vi "DefineVariableChoice.vi"() -> ()   [LabVIEW 2020]
panel:
  in  "Set":bool
  in  "Exit":bool
  in  "Add Choices":string
  in  "Choices":u16(ring) items=["numeric", "string", "1darray", "image", "on,off", "open,closed", "low,medium,high", "path", "outofrange,inrange", "1 mega ohm,50 ohms", "AC,DC,Ground", "Positive,Negative", "Field 1,Field2,Any Field,Any Line,Any Number", "AC,DC,HF Reject,LF Reject,AC Plus HF Reject", "Channel 0,Channel 1,External TRIG", "Entering,Leaving", "M-NTSC,B/G-PAL,SECAM,M-PAL,more", "Immediate,Analog Edge,Analog Window,Analog Hysteresis,Video,Digital Edge", "T0,T1,A,B,C,D,E,F,G,H", "Internal,External rising edges,External falling edges,Single shot external rising edges,Single shot external falling edges,Single shot,Line", "off,Triggers,AB,AB and CD,AB, CD and EF,AB, CD, EF and GH", "off,1,2,3,4,5,6,7,8,9", "T0,B,C,D", "T0,A,C,D", "T0,A,B,D", "T0,A,B,C", "TCPIP,Serial", "Not referenced,Referenced", "MZ switch and encoder Index,current position as HOME,MZ switch only,EoR- switch and encoder Index,EoR- switch only", "NOT REFERENCED,CONFIGURATION,HOMING,MOVING,READY,DISABLE,JOGGING", "High Z,50 Ohm", "TTL,NIM,ECL,VAR", "Internal,External,Single Shot,Burst,Line", "+ve edge,-ve edge", "Not referenced,Homing,Moving,Ready", "RTSI 0,RTSI 1,RTSI 2,RTSI 3,RTSI 4,RTSI 5,RTSI 6,PFI 0,PFI 1,PFI 2,PXI Star Trigger", "Continuous,Single Shot", "Not referenced,Homing,Moving,Ready", "Forward,Backward,Undefined", "pos,neg", "1,2,4,5,10", "TTL0,TTL1,TTL2,TTL3,TTL4,TTL5,TTL6,TTL7,ECL0,ECL1,Input Channel 1,Input Channel 2,Input Channel 3,Input Channel 4,External Trigger Source,STAR,Manual Trigger,Pattern", "1,2,3,4,5,6", "Diode,Low Power,High Power,undefined", "Error,Moving,OK", "n/a,max,min,energy", "Flipper,Plunger", "Remove,Insert", "IN,OUT", "Internal,External", "1f,3f,10f,30f,100f,300f,1p,3p,10p,30p,100p,300p,1n,3n,10n,30n,100n,300n,1u,3u,10u,30u,100u,300u,1m,3m,10m,30m,100m,300m,1,3,10,30,100,300,1k,3k,10k,30k,100k,300k,1M,3M,10M,30M,100M,300M", "yes,no", "IS_SET_TRIG_OFF,IS_SET_TRIG_HI_LO,IS_SET_TRIG_LO_HI,IS_SET_TRIG_SOFTWARE,IS_GET_EXTERNAL_TRIGGER,IS_GET_TRIGGER_STATUS", "Disable,High,Low", "64,128,256,512", "Moving/Unknown,OD1,OD2,OD3,OD4,OD5,Open(6)", "temporal CAM,spatial CAM", "out,in,Unknown", "Channel0,Channel1,Channel2,Channel3,Channel4,Channel5,Channel6,Channel7,n/a", "n/a,max,min,energy,trigger,maxtime,mintime,mean", "absolute,gauge", "1p,3p,10p,30p,100p,300p,1n,3n,10n,30n,100n,300n,1u,3u,10u,30u,100u,300u,1m,3m,10m,30m,100m,300m,1,3,10,30,100,300,1k,3k,10k,30k,100k,300k,1meg,3meg,10meg,30meg,100meg,300meg", "Internal 1,Internal 2,External,SS1,SS2,SSExt,LSS,OFF", "off,on,reset,fault", "Double,Boolean", "n/a,max,min,energy,trigger,maxtime,mintime,mean", "FL1-f8x08,FL1-f8x06,FL1-f8,ch300-f50,FL2G-f8,FL3M14-f8,FL3M14-f8x08,FL3M14-f8x08(2x2)", "Serial,TCP", "Pressure,Flow", "Numeric,String", "N/A,Free Run/Timed,Trigger First (PM only),Ext Sync/Strobed,Variable Exp (PM only),Flash Mode (PM only)", "Software,Hardware", "Immediate,Analog Edge", "Channel1,Channel2,Channel3,Channel4,AC Line,Aux", "DC,HF Reject,LF Reject,Noise Reject,AC", "Rising,Falling", "1E+3,10E+3,100E+3,1E+6,5E+6,10E+6", "1M,75,50", "FULL,250 MHz, 150 MHz, 20 MHz", "Channel 1,Channel 2,Channel 3,Channel 4,Math,Reference 1,Reference 2,Reference 3,Reference 4,Bus 1,Bus 2", "10KOhm,50Ohms", "Rising,Falling,Internal 80Mhz,Internal DSS,Remote,Disable", "Direct,Inverted", "Null,A,B,C,D,Trigger", "Auto,Manual", "J,K,N,R,S,T,B,E", "Deg C,Deg F,Kelvins,Deg R,From Custom Scale", "Built-In,Constant Value,Channel", "1f,3f,10f,30f,100f,300f,1p,3p,10p,30p,100p,300p,1n,3n,10n,30n,100n,300n,1u,3u,10u,30u,100u,300u,1m,3m,10m,30m,100m,300m,1,3,10,30,100,300,1K,3K,10K,30K,100K,300K,1M,3M,10M,30M,100M,300M", "left,right", "on demand,continuous,scan", "1,2,3,4", "50,100,250,500,1000,2500,5K,10K,25K,50K,100K,250K,500K,1M,2M,2.5M,5M,10M,25M,50M,100M", "Full,20MHZ,25MHZ,200MHZ,250MHZ,1GHZ,3GHZ,4GHZ", "Channel 1,Channel 2,Channel 3,Channel 4,External,Power Line", "Auto,Normal,Single,Single, auto trigger", "A1M,D1M,D50,Ground,DC,AC", "POS (+),NEG (-)", "HOME,POS (+),NEG (-)", "Idel,Moving,L- (neg limit),L+ (pos limit),Homed", "HOME,POS (+),NEG (-),none", "HOME,POS (+),NEG (-),done", "Full,20MHZ,200MHZ", "Full,25MHZ,20MHZ,200MHZ", "HOME,done", "Idel,Moving,Accelerating,Decelerating,L- (neg limit),L+ (pos limit),Homed", "homing,limiting,done", "true,false", "default,inverted", "choice", "Enable,Disable", "4J,8J", "50usec,100usec", "Energy,Power", "Removed,Inserted,Unknown,Moving", "20.00J,4.00J,400mJ,40.0mJ,4.00mJ", "50uS,1.0mS", "248,355,532,800,2940,193", "Auto,Normal,Single,Single auto trigger", "Voltage,Current", "PNG,BMP,JPEG,TDMS", "PNG,BMP,JPEG,TDMS,hdf5", "FL1-f8x08,FL1-f8x06,FL1-f8,ch300-f50,FL2G-f8,FL3M14-f8,FL3M14-f8x08,FL3M14-f8x08(2x2),aca720-f8,aca1440-f8", "10 mV, 20mV, 50mV, 100mV, 200mV, 500mV, 1V, 2V, 5V, 10V, 20V"]
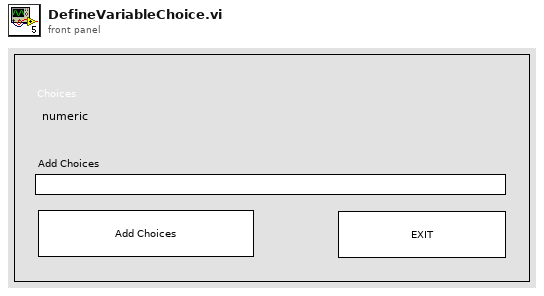
[diagram p1: front panel]
types:
  T1 = enum32{"Invalid", "Standard", "Closed", "Hidden", "Minimized", "Maximized"}
  T2 = enum32{"invalid app kind", "Development System", "Run Time System", "Student Edition", "Embedded LabVIEW", "Evaluation", "Custom"}
  T3 = typedef "mysql_authentication.ctl" = cluster{"User":string, "Password":string, "Database":string}
  T4 = cluster{"Core":cluster{"Current VI Reference":refnum<vi>, "Close Panel on Exit?":bool}, "SQL Server Info":cluster{"Port":u16, "IP Address":string, "Authentication":T3}, "Your string data":string}
  T5 = cluster{"Port":u16, "IP Address":string, "Authentication":T3}
  T6 = cluster{"Current VI Reference":refnum<vi>, "Close Panel on Exit?":bool}
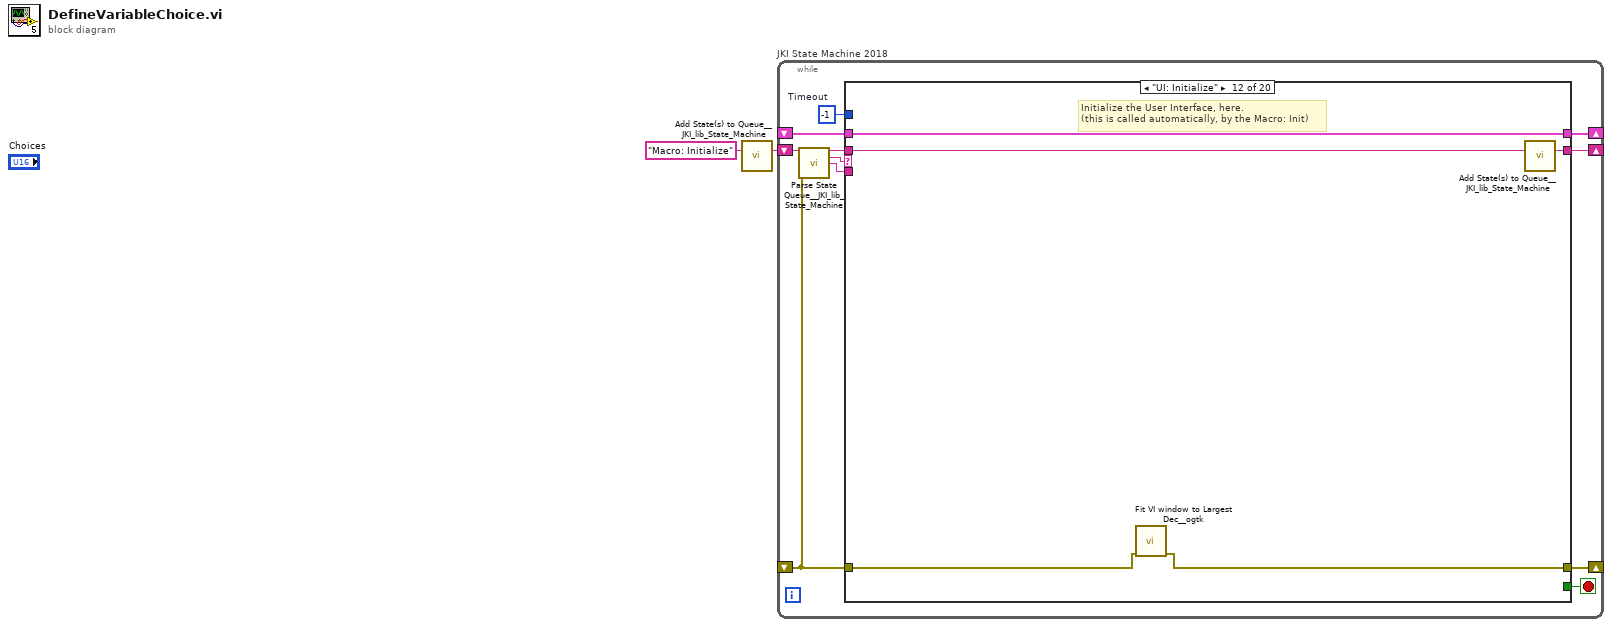
[diagram p0: block diagram]
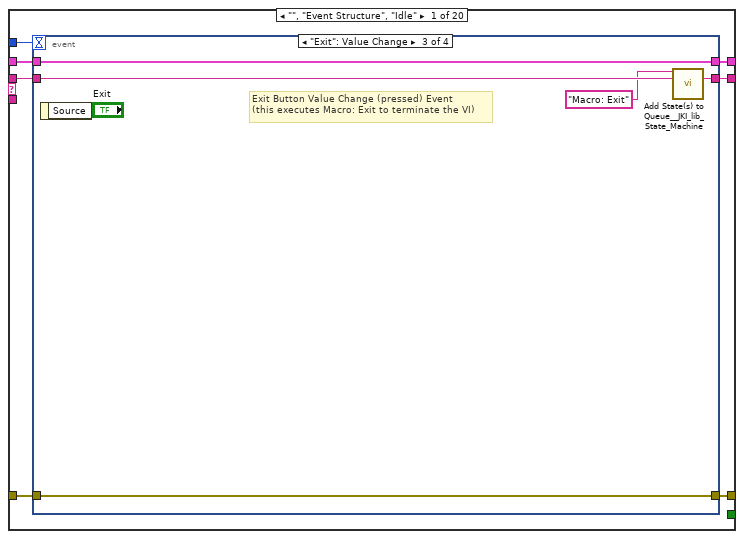
[diagram p2: hidden frame]
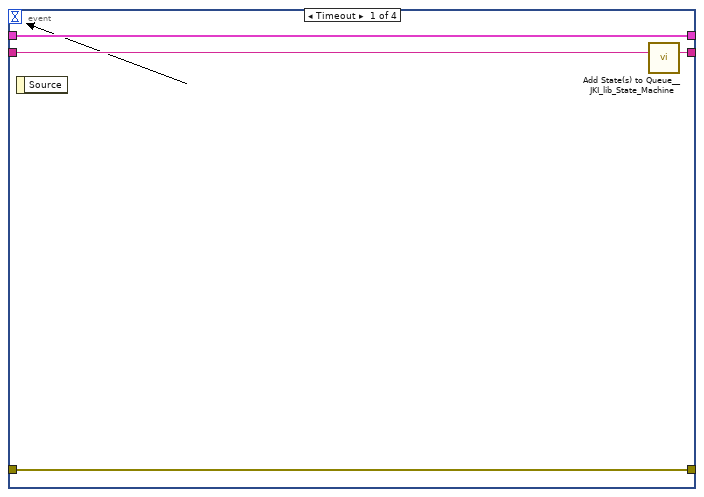
[diagram p3: hidden frame]
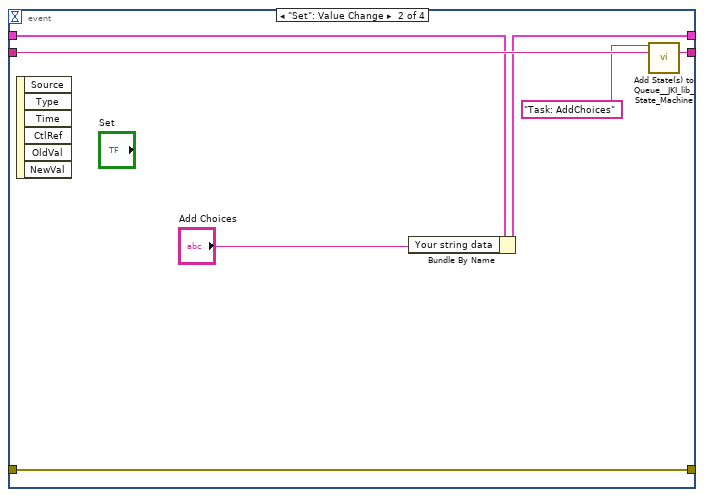
[diagram p4: hidden frame]
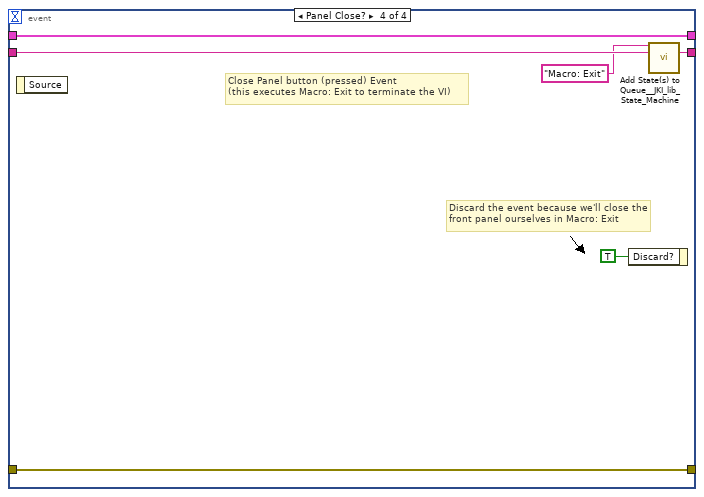
[diagram p5: hidden frame]
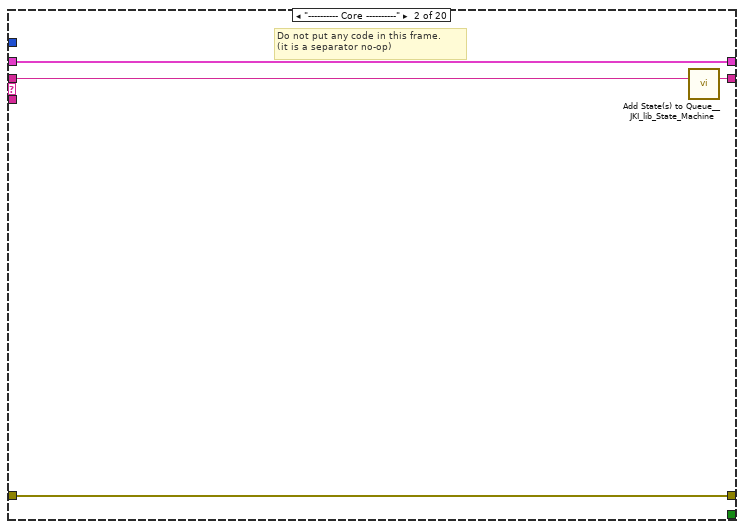
[diagram p6: hidden frame]
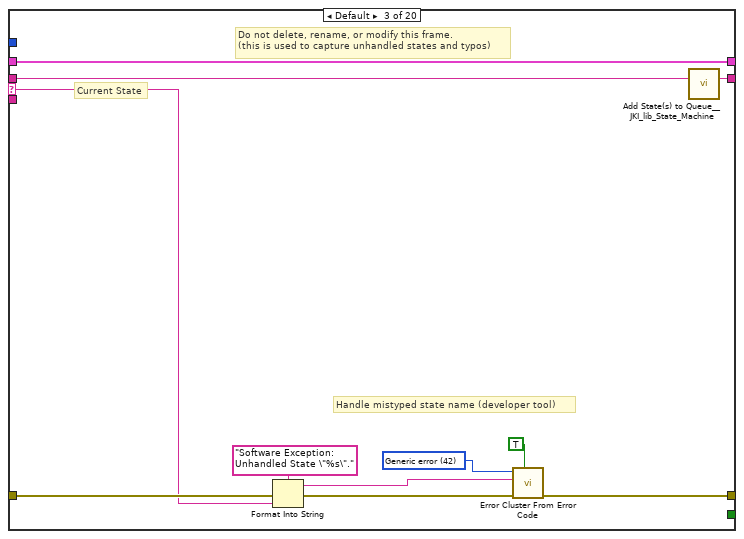
[diagram p7: hidden frame]
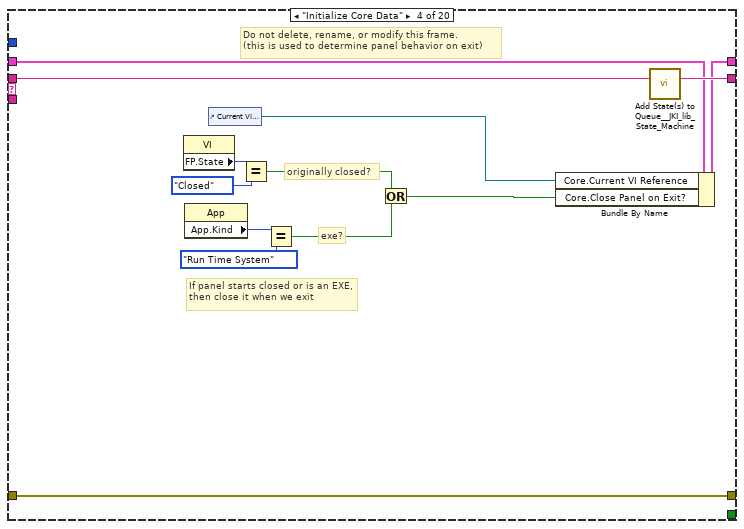
[diagram p8: hidden frame]
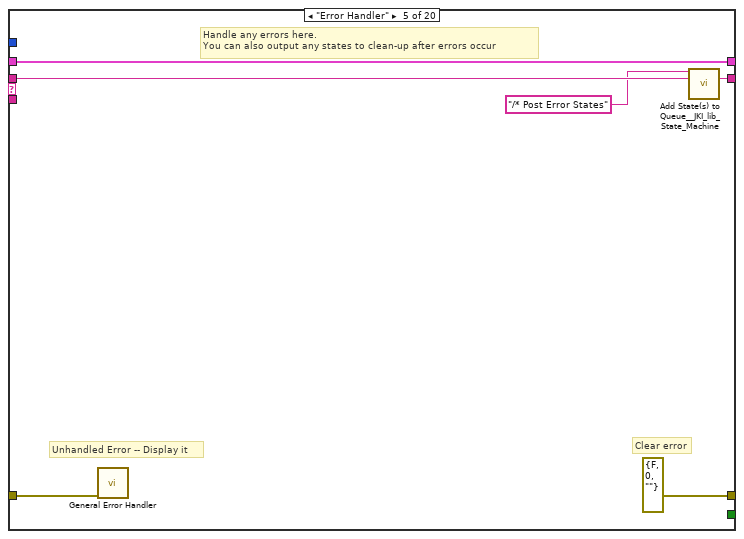
[diagram p9: hidden frame]
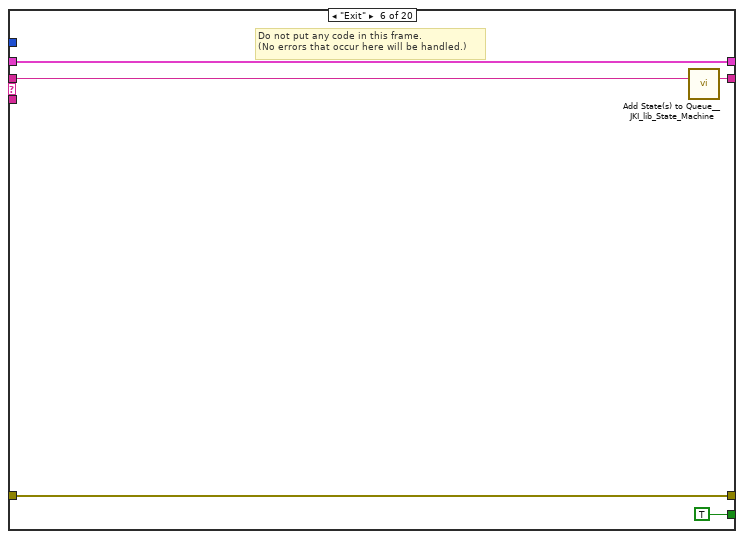
[diagram p10: hidden frame]
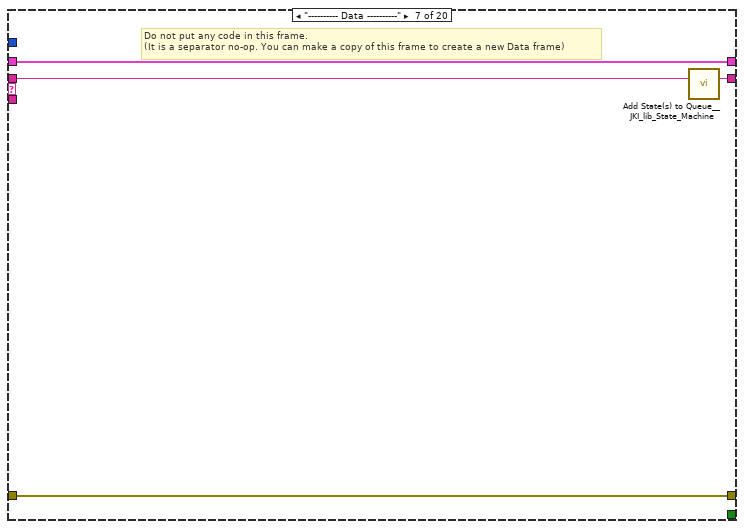
[diagram p11: hidden frame]
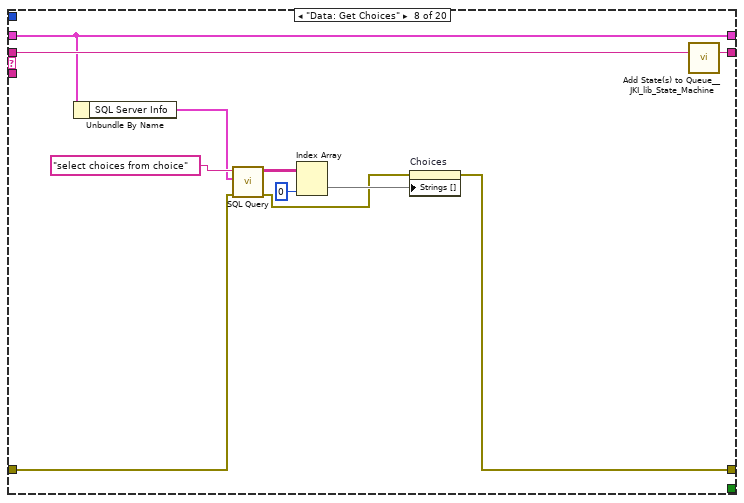
[diagram p12: hidden frame]
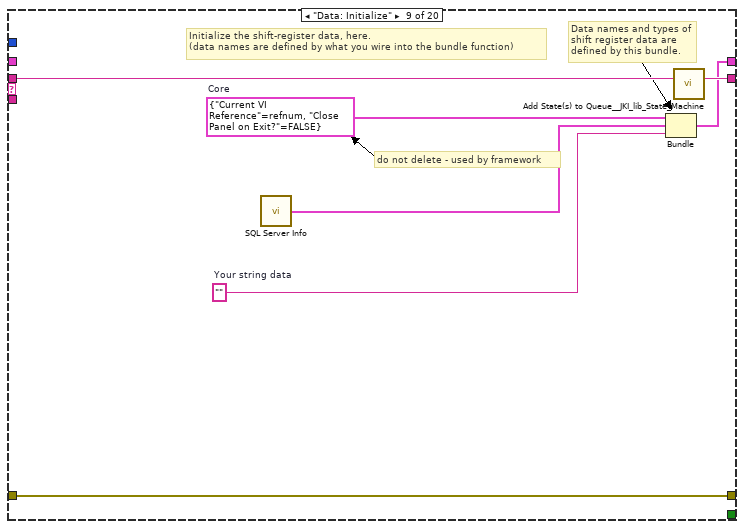
[diagram p13: hidden frame]
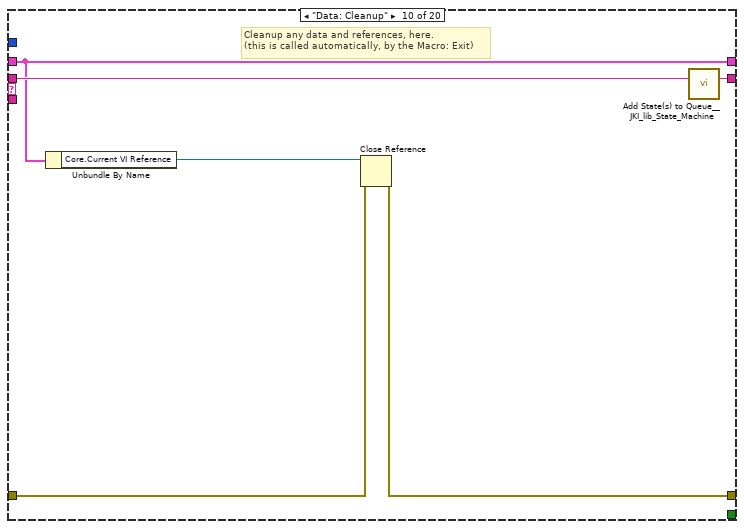
[diagram p14: hidden frame]
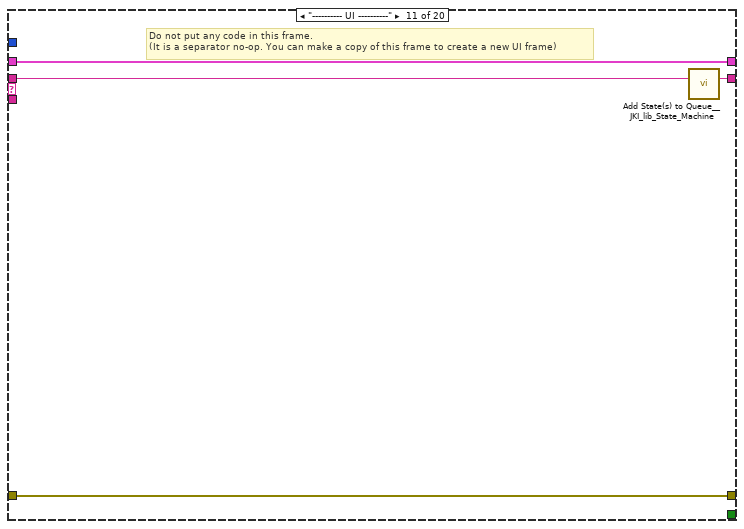
[diagram p15: hidden frame]
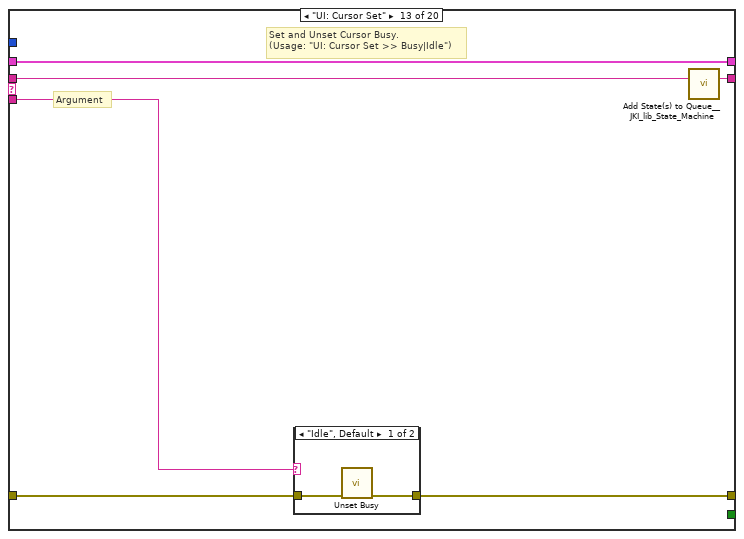
[diagram p16: hidden frame]
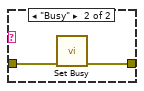
[diagram p17: hidden frame]
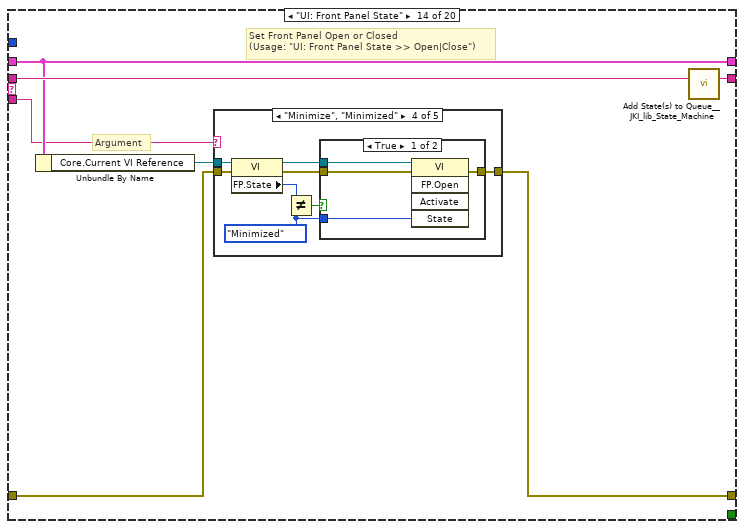
[diagram p18: hidden frame]
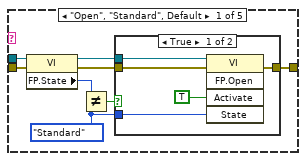
[diagram p19: hidden frame]
diagram:
  n1 = call <vilib>:"Add State(s) to Queue__JKI_lib_State_Machine.vi"("State(s) in (\"\")"="Macro: Initialize") -> ("States Out"=w2:string)  [unwired: 14 in]
  n2 = while "JKI State Machine 2018" {
    shift-right: [w6] -> _
    shift-left: _ -> [w5]
    shift-right: [w9] -> _
    shift-left: _ -> [w3]
    shift-right: [w8] -> _
    shift-left: w2 -> [w10]
    stop <- w7 stop-if-true
    w4 = -1  # Timeout
    n3 = call <vilib>:"Parse State Queue__JKI_lib_State_Machine.vi"("State Queue"=w10, "Error In (no error)"=w3) -> ("Remaining States"=w12:string, "Current State"=w13:string, "Arguments"=w11:string)  [unwired: 11 in]
    n4 = case shown="\"UI: Initialize\"" w13 {
      selector: w13 -> [_ _ w47 _ _ _ _ _ _ _ _ _ _ _ _ _ _ _ _ _]
      tunnel: w12 -> [w20 w46 w51 w70 w76 w81 w85 w96 w103 w109 w113 w118 w124 w135 w204 w209 w219 w223 w234 w238]
      tunnel: w11 -> [_ _ _ _ _ _ _ _ _ _ _ _ w119 w129 _ _ _ _ _ _]
      tunnel: w5 -> [w18 w43 w49 w63 w73 w79 w82 w94 _ w104 w110 w116 w122 w131 w201 w206 w216 w220 w229 w235]
      tunnel: [w17 w44 w53 w67 errorcluster {"status"=FALSE, "code"=0, "source"=""} ("error out") w78 w83 w86 w100 w105 w111 w115 w120 w132 w202 w207 w217 w221 w225 w236] -> w9
      tunnel: w3 -> [w16 w44 w52 w67 w72 w78 w83 w88 w100 w106 w111 w114 w121 w133 w202 w207 w217 w221 w224 w236]
      tunnel: [w19 w45 w50 w69 w75 w80 w84 w95 w102 w108 w112 w117 w123 w134 w203 w208 w218 w222 w233 w237] -> w8
      tunnel: [_ _ _ _ _ TRUE _ _ _ _ _ _ _ _ _ _ _ _ _ _] -> w7
      tunnel: [w15 w43 w49 w68 w73 w79 w82 w94 w101 w104 w110 w116 w122 w131 w201 w206 w216 w220 w229 w235] -> w6
      tunnel: w4 -> [w14 _ _ _ _ _ _ _ _ _ _ _ _ _ _ _ _ _ _ _]
      frame "", "Event Structure", "Idle" {
        n5 = event shown="[2] \"Exit\": Value Change" {
          selector: _ -> [_ _ _ _]
          dyn-events: _ -> [_ _ _ _]
          timeout: w14 -> [_ _ _ _]
          tunnel: w20 -> [w24 w31 w36 w42]
          tunnel: [w23 w30 w35 w41] -> w19
          tunnel: w18 -> [w21 w28 w33 w39]
          tunnel: [w22 w29 w34 w40] -> w17
          tunnel: w16 -> [w22 w29 w34 w40]
          tunnel: [w21 w27 w33 w39] -> w15
          event Timeout {
            n6 = event-data() -> ()  [unwired: 1 in, 1 out]
            n7 = call <vilib>:"Add State(s) to Queue__JKI_lib_State_Machine.vi"("State(s) in (\"\")"=w24) -> ("States Out"=w23:string)  [unwired: 14 in]
          }
          event "Set": Value Change {
            n8 = event-data() -> ()  [unwired: 1 in, 6 out]
            n9 = Bundle By Name(cluster=w28, "Your string data"="Add Choices") -> (w27:T4)
            n10 = call <vilib>:"Add State(s) to Queue__JKI_lib_State_Machine.vi"("State(s) in Front (\"\")"="Task: AddChoices" ("State(s) in Front (\"\")"), "State(s) in (\"\")"=w31) -> ("States Out"=w30:string)  [unwired: 13 in]
          }
          event "Exit": Value Change {
            # "Exit Button Value Change (pressed) Event\n(this executes Macro: Exit to terminate the VI)"
            n11 = event-data() -> ()  [unwired: 1 in, 1 out]
            n12 = call <vilib>:"Add State(s) to Queue__JKI_lib_State_Machine.vi"("State(s) in Front (\"\")"="Macro: Exit", "State(s) in (\"\")"=w36) -> ("States Out"=w35:string)  [unwired: 13 in]
          }
          event Panel Close? {
            # "Discard the event because we'll close the front panel ourselves in Macro: Exit"
            # "Close Panel button (pressed) Event\n(this executes Macro: Exit to terminate the VI)"
            n13 = event-data() -> ()  [unwired: 1 in, 1 out]
            n14 = event-data("Discard?"=TRUE) -> ()  [unwired: 1 in, 1 out]
            n15 = call <vilib>:"Add State(s) to Queue__JKI_lib_State_Machine.vi"("State(s) in Front (\"\")"="Macro: Exit", "State(s) in (\"\")"=w42) -> ("States Out"=w41:string)  [unwired: 13 in]
          }
        }
      }
      frame "---------- Core ----------" {
        # "Do not put any code in this frame.\n(it is a separator no-op)"
        n16 = call <vilib>:"Add State(s) to Queue__JKI_lib_State_Machine.vi"("State(s) in (\"\")"=w46) -> ("States Out"=w45:string)  [unwired: 14 in]
      }
      frame Default {
        w56 = 42 items=["No error", "Argument error", "Memory is full", "Out of zone", "End of file", "File already open", "Generic file I/O error", "File not found", "File permission error", "Disk is full", "Duplicate path", "Too many files open", "System feature not enabled", "Resource file not found", "Cannot add resource", "Resource not found", "Image not found", "Image memory error", "Pen does not exist", "Config type invalid", "Config token not found", "Config parse error", "Config memory error", "Bad external code format", "Bad external code offset", "External code not present", "Null window", "Destroy window error", "Null menu", "Print aborted", "Bad print record", "Print driver error", "Windows error during printing", "Memory error during printing", "Print dialog error", "Generic print error", "Invalid device refnum", "Device not found", "Device parameter error", "Device unit error", "Cannot open device", "Device call aborted", "Generic error", "Cancelled by user", "Object ID too low", "Object ID too high", "Object not in heap", "Unknown heap", "Unknown object (invalid DefProc)", "Unknown object (DefProc not in table)", "Message out of range", "Invalid (null) method", "Unknown message", "Manager call not supported", "Bad address", "Network operation in progress", "Network operation timed out", "Connection is busy", "Network attribute not supported", "Network error", "Address in use", "System out of memory", "Connection aborted", "Connection refused", "Not connected", "Already connected", "Connection closed", "Initialization error (interapplication manager)", "Bad occurrence", "Wait on unbound occurrence handler", "Occurrence queue overflow", "Datalog type conflict", "Unused", "Unrecognized type (interapplication manager)", "Memory corrupt", "Failed to make temporary DLL", "Old CIN version", "Drag socket not found", "Failed to load drop-object", "Failed to register OLE object", "Failed to release OLE object", "Format specifier type mismatch", "Unknown format specifier", "Too few format specifiers", "Too many format specifiers", "Scan failed", "Newer CIN version", "Error converting to variant", "Runtime menu error", "Password tampered", "Variant attribute not found", "Incompatible variant data type", "Event data is not available", "Event Store is not present", "Occurrence is not found", "Event Queue is not created", "Event info is not available", "Refnum passed is NULL", "Error retrieving Class GUID", "Error retrieving CoClass GUID", "Error retrieving TypeLib GUID.", "Bad built application magic bytes.", "Specific driver is different from the specific driver associated with the Logical Name.", "There is no session opened to the class driver.", "Max Error", "MAX - Error with config objects", "MAX - Error loading configuration", "MAX - Group not supported"]
        # "Current State"
        # "Do not delete, rename, or modify this frame.\n(this is used to capture unhandled states and typos)"
        # "Handle mistyped state name (developer tool)"
        n17 = Format Into String(format string="Software Exception: Unhandled State \"%s\"." ("message"), error in=w52, w47) -> (resulting string=w55:string, error out=w54:errorcluster)  [unwired: 1 in]
        n18 = call <vilib>:"Error Cluster From Error Code.vi"("show call chain? (False)"=TRUE, "error in (no error)"=w54, "error message (\"\")"=w55, "error code (0)"=w56) -> ("error out"=w53:errorcluster)  [unwired: 5 in]
        n19 = call <vilib>:"Add State(s) to Queue__JKI_lib_State_Machine.vi"("State(s) in (\"\")"=w51) -> ("States Out"=w50:string)  [unwired: 14 in]
      }
      frame "Initialize Core Data" {
        # "Do not delete, rename, or modify this frame.\n(this is used to determine panel behavior on exit)"
        # "originally closed?"
        # "exe?"
        # "If panel starts closed or is an EXE, then close it when we exit"
        n20 = property class="VI"() -> ("FP.State"=w60:T1)  [unwired: 2 in, 2 out]
        n21 = property class="App"() -> ("App.Kind"=w66:T2)  [unwired: 2 in, 2 out]
        n22 = control-ref of="Current VI Reference"() -> (w61:refnum<vi>)
        n23 = Equal?(x=w60, y=T1."Closed" ("Front Panel Window:State")) -> (x = y?=w58:bool)
        n24 = Equal?(x=w66, y=T2."Run Time System" ("Application:Kind")) -> (x = y?=w64:bool)
        n25 = Or(x=w58, y=w64) -> (x .or. y?=w62:bool)
        n26 = Bundle By Name(cluster=w63, "Core.Current VI Reference"=w61, "Core.Close Panel on Exit?"=w62) -> (w68:T4)
        n27 = call <vilib>:"Add State(s) to Queue__JKI_lib_State_Machine.vi"("State(s) in (\"\")"=w70) -> ("States Out"=w69:string)  [unwired: 14 in]
      }
      frame "Error Handler" {
        # "Unhandled Error -- Display it"
        # "Handle any errors here.\nYou can also output any states to clean-up after errors occur"
        # "Clear error"
        n28 = call <vilib>:"General Error Handler.vi"("error in (no error)"=w72) -> ()  [unwired: 10 in, 5 out]
        n29 = call <vilib>:"Add State(s) to Queue__JKI_lib_State_Machine.vi"("State(s) in Front (\"\")"="/* Post Error States", "State(s) in (\"\")"=w76) -> ("States Out"=w75:string)  [unwired: 13 in]
      }
      frame "Exit" {
        # "Do not put any code in this frame.\n(No errors that occur here will be handled.)"
        n30 = call <vilib>:"Add State(s) to Queue__JKI_lib_State_Machine.vi"("State(s) in (\"\")"=w81) -> ("States Out"=w80:string)  [unwired: 14 in]
      }
      frame "---------- Data ----------" {
        # "Do not put any code in this frame.\n(It is a separator no-op. You can make a copy of this frame to create a new Data frame)"
        n31 = call <vilib>:"Add State(s) to Queue__JKI_lib_State_Machine.vi"("State(s) in (\"\")"=w85) -> ("States Out"=w84:string)  [unwired: 14 in]
      }
      frame "Data: Get Choices" {
        n32 = Unbundle By Name(w94) -> ("SQL Server Info"=w89:T5)
        n33 = call "SQL Query.vi"("error in (no error)"=w88, "SQL Server Info"=w89, "Query"="select choices from choice") -> ("error out"=w87:errorcluster, "data"=w92:string[][])  [unwired: 7 in]
        n34 = Index Array(array=w92, index (col)=0 ("disabled index (col)")) -> (element=w93:string[])  [unwired: 1 in]
        n35 = property on="Choices" class="Ring (strict)"(error in=w87, "Strings []"=w93) -> (error out=w86:errorcluster)  [unwired: 1 in, 1 out]
        n36 = call <vilib>:"Add State(s) to Queue__JKI_lib_State_Machine.vi"("State(s) in (\"\")"=w96) -> ("States Out"=w95:string)  [unwired: 14 in]
      }
      frame "Data: Initialize" {
        w98 = T6 {"Current VI Reference"=refnum, "Close Panel on Exit?"=FALSE}  # Core
        w99 = ""  # Your string data
        # "do not delete - used by framework"
        # "Data names and types of shift register data are defined by this bundle."
        # "Initialize the shift-register data, here.\n(data names are defined by what you wire into the bundle function)"
        n37 = call "SQL Server Info.vi"() -> ("SQL Server Info"=w97:T5)
        n38 = Bundle("Core"=w98, "SQL Server Info"=w97, "Your string data"=w99) -> (w101:T4)  [unwired: 1 in]
        n39 = call <vilib>:"Add State(s) to Queue__JKI_lib_State_Machine.vi"("State(s) in (\"\")"=w103) -> ("States Out"=w102:string)  [unwired: 14 in]
      }
      frame "Data: Cleanup" {
        # "Cleanup any data and references, here.\n(this is called automatically, by the Macro: Exit)"
        n40 = Unbundle By Name(w104) -> ("Core.Current VI Reference"=w107:refnum<vi>)
        n41 = Close Reference(reference=w107, error in (no error)=w106) -> (error out=w105:errorcluster)
        n42 = call <vilib>:"Add State(s) to Queue__JKI_lib_State_Machine.vi"("State(s) in (\"\")"=w109) -> ("States Out"=w108:string)  [unwired: 14 in]
      }
      frame "---------- UI ----------" {
        # "Do not put any code in this frame.\n(It is a separator no-op. You can make a copy of this frame to create a new UI frame)"
        n43 = call <vilib>:"Add State(s) to Queue__JKI_lib_State_Machine.vi"("State(s) in (\"\")"=w113) -> ("States Out"=w112:string)  [unwired: 14 in]
      }
      frame "UI: Initialize" {
        # "Initialize the User Interface, here.\n(this is called automatically, by the Macro: Init)"
        n44 = call <userlib>:"Fit VI window to Largest Dec__ogtk.vi"("error in (no error)"=w114) -> ("error out"=w115:errorcluster)  [unwired: 5 in, 1 out]
        n45 = call <vilib>:"Add State(s) to Queue__JKI_lib_State_Machine.vi"("State(s) in (\"\")"=w118) -> ("States Out"=w117:string)  [unwired: 14 in]
      }
      frame "UI: Cursor Set" {
        # "Argument"
        # "Set and Unset Cursor Busy.\n(Usage: \"UI: Cursor Set >> Busy|Idle\")"
        n46 = case shown="\"Idle\", Default" w119 {
          tunnel: w121 -> [w126 w128]
          tunnel: [w125 w127] -> w120
          frame "Idle", Default {
            n47 = call <vilib>:"Unset Busy.vi"("error in (no error)"=w126) -> ("error out"=w125:errorcluster)  [unwired: 10 in]
          }
          frame "Busy" {
            n48 = call <vilib>:"Set Busy.vi"("error in (no error)"=w128) -> ("error out"=w127:errorcluster)  [unwired: 9 in, 1 out]
          }
        }
        n49 = call <vilib>:"Add State(s) to Queue__JKI_lib_State_Machine.vi"("State(s) in (\"\")"=w124) -> ("States Out"=w123:string)  [unwired: 14 in]
      }
      frame "UI: Front Panel State" {
        # "Argument"
        # "Set Front Panel Open or Closed\n(Usage: \"UI: Front Panel State >> Open|Close\")"
        n50 = Unbundle By Name(w131) -> ("Core.Current VI Reference"=w130:refnum<vi>)
        n51 = case shown="\"Minimize\", \"Minimized\"" w129 {
          tunnel: w133 -> [w141 w156 w167 w180 w193]
          tunnel: [w143 w157 w169 w182 w195] -> w132
          tunnel: w130 -> [w142 w154 w168 w181 w194]
          frame "Open", "Standard", Default {
            w136 = T1."Standard" ("State")
            n52 = property class="VI"(reference=w142, error in=w141) -> (reference out=w139:refnum<vi>, error out=w140:errorcluster, "FP.State"=w138:T1)
            n53 = Not Equal?(x=w138, y=w136) -> (x != y?=w137:bool)
            n54 = case shown="True" w137 {
              tunnel: [w147 w149] -> w143
              tunnel: w140 -> [w146 w149]
              tunnel: w139 -> [w145 _]
              tunnel: w136 -> [w144 _]
              frame True {
                n55 = invoke class="VI" method="FP.Open"(reference=w145, error in=w146, "Activate"=TRUE, "State"=w144) -> (error out=w147:errorcluster)  [unwired: 1 in, 4 out]
              }
              frame False {
              }
            }
          }
          frame "Close", "Closed" {
            n56 = property class="VI"(reference=w154, error in=w156) -> (reference out=w153:refnum<vi>, error out=w155:errorcluster, "FP.State"=w151:T1)
            n57 = Not Equal?(x=w151, y=T1."Closed" ("Front Panel Window:State")) -> (x != y?=w150:bool)
            n58 = case shown="True" w150 {
              tunnel: [w158 w161] -> w157
              tunnel: w155 -> [w158 w160]
              tunnel: w153 -> [_ w159]
              frame False {
              }
              frame True {
                n59 = invoke class="VI" method="FP.Close"(reference=w159, error in=w160) -> (error out=w161:errorcluster)  [unwired: 1 in, 2 out]
              }
            }
          }
          frame "Hidden", "Hide" {
            w162 = T1."Hidden" ("State")
            n60 = property class="VI"(reference=w168, error in=w167) -> (reference out=w165:refnum<vi>, error out=w166:errorcluster, "FP.State"=w164:T1)
            n61 = Not Equal?(x=w164, y=w162) -> (x != y?=w163:bool)
            n62 = case shown="True" w163 {
              tunnel: [w173 w174] -> w169
              tunnel: w166 -> [w172 w174]
              tunnel: w165 -> [w171 _]
              tunnel: w162 -> [w170 _]
              frame True {
                n63 = invoke class="VI" method="FP.Open"(reference=w171, error in=w172, "State"=w170) -> (error out=w173:errorcluster)  [unwired: 2 in, 4 out]
              }
              frame False {
              }
            }
          }
          frame "Minimize", "Minimized" {
            w175 = T1."Minimized" ("State")
            n64 = property class="VI"(reference=w181, error in=w180) -> (reference out=w178:refnum<vi>, error out=w179:errorcluster, "FP.State"=w177:T1)
            n65 = Not Equal?(x=w177, y=w175) -> (x != y?=w176:bool)
            n66 = case shown="True" w176 {
              tunnel: [w186 w187] -> w182
              tunnel: w179 -> [w185 w187]
              tunnel: w178 -> [w184 _]
              tunnel: w175 -> [w183 _]
              frame True {
                n67 = invoke class="VI" method="FP.Open"(reference=w184, error in=w185, "State"=w183) -> (error out=w186:errorcluster)  [unwired: 2 in, 4 out]
              }
              frame False {
              }
            }
          }
          frame "Maximize", "Maximized" {
            w188 = T1."Maximized" ("State")
            n68 = property class="VI"(reference=w194, error in=w193) -> (reference out=w191:refnum<vi>, error out=w192:errorcluster, "FP.State"=w190:T1)
            n69 = Not Equal?(x=w190, y=w188) -> (x != y?=w189:bool)
            n70 = case shown="True" w189 {
              tunnel: [w199 w200] -> w195
              tunnel: w192 -> [w198 w200]
              tunnel: w191 -> [w197 _]
              tunnel: w188 -> [w196 _]
              frame True {
                n71 = invoke class="VI" method="FP.Open"(reference=w197, error in=w198, "State"=w196) -> (error out=w199:errorcluster)  [unwired: 2 in, 4 out]
              }
              frame False {
              }
            }
          }
        }
        n72 = call <vilib>:"Add State(s) to Queue__JKI_lib_State_Machine.vi"("State(s) in (\"\")"=w135) -> ("States Out"=w134:string)  [unwired: 14 in]
      }
      frame "---------- Macro ----------" {
        # "Do not put any code in this frame.\n(It is a separator no-op. You can make a copy of this frame to create a new Macro frame)"
        n73 = call <vilib>:"Add State(s) to Queue__JKI_lib_State_Machine.vi"("State(s) in (\"\")"=w204) -> ("States Out"=w203:string)  [unwired: 14 in]
      }
      frame "Macro: Initialize" {
        w205 = "Data: Initialize\nInitialize Core Data\nUI: Initialize\nUI: Front Panel State >> Open\nData: Get Choices"  # Data: Initialize Initialize Core Data UI: Initialize UI: Front Panel State >> Open Data: Get Choices
        # "Initialization Macro\n(This is called once, when the VI starts)"
        n74 = call <vilib>:"Add State(s) to Queue__JKI_lib_State_Machine.vi"("State(s) in Front (\"\")"=w205, "State(s) in (\"\")"=w209) -> ("States Out"=w208:string)  [unwired: 13 in]
      }
      frame "Macro: Exit" {
        # "Exit Macro\n(This is called once, when the VI exits)"
        n75 = Unbundle By Name(w216) -> ("Core.Close Panel on Exit?"=w215:bool)
        n76 = Select(t="UI: Front Panel State >> Close", s=w215, f="") -> (s? t:f=w212:string)
        n77 = call <vilib>:"Add State(s) to Queue__JKI_lib_State_Machine.vi"("State(s) in (\"\")"=w212, "State(s) at Back (\"\")"="Data: Cleanup\nExit") -> ("States Out"=w210:string)  [unwired: 13 in]
        n78 = call <vilib>:"Add State(s) to Queue__JKI_lib_State_Machine.vi"("State(s) in Front (\"\")"=w210, "State(s) in (\"\")"=w219) -> ("States Out"=w218:string)  [unwired: 13 in]
      }
      frame "---------- Task ----------" {
        # "Template Separator\n(You can make a copy of, or modify, this frame)"
        n79 = call <vilib>:"Add State(s) to Queue__JKI_lib_State_Machine.vi"("State(s) in (\"\")"=w223) -> ("States Out"=w222:string)  [unwired: 14 in]
      }
      frame "Task: AddChoices" {
        n80 = Unbundle By Name(w229) -> ("Your string data"=w228:string, "SQL Server Info"=w226:T5)
        n81 = Build Array(w228) -> (w227:string[])
        n82 = call "SQL Insert.vi"("Values"=w227, "Column Names"=string[] ["choices"], "Table"="choice") -> ("Query String"=w232:string)  [unwired: 8 in]
        n83 = call "SQL Query.vi"("error in (no error)"=w224, "SQL Server Info"=w226, "Query"=w232) -> ("error out"=w225:errorcluster)  [unwired: 7 in, 1 out]
        n84 = call <vilib>:"Add State(s) to Queue__JKI_lib_State_Machine.vi"("State(s) in (\"\")"=w234) -> ("States Out"=w233:string)  [unwired: 14 in]
      }
      frame "New Category: 2" {
        # "Your code here.\n(You can make a copy of, or modify, this frame)"
        n85 = call <vilib>:"Add State(s) to Queue__JKI_lib_State_Machine.vi"("State(s) in (\"\")"=w238) -> ("States Out"=w237:string)  [unwired: 14 in]
      }
    }
  }
